vi "MB Serial Master Query Read HF.vi"(8 "error in":errorcluster, 10 "Set Points":dbl[](array[numeric])=[1.0], 11 "VISA resource name":refnum<visa-resource-name>) -> (0 "error out":errorcluster, 2 "Meter reading":sgl, 3 "VISA resource name out":refnum<visa-resource-name>, 5 "Unit id":i32)   [LabVIEW 2015]
doc: "The master uses this VI to read the slaves input registers. This corresponds to a public function code of 4 in the MODBUS protocol."
uses:
  MB Modbus Command.ctl
panel:
  out "Exception Code":u8 format="%.0x"
  in  "Timeout":u32=500
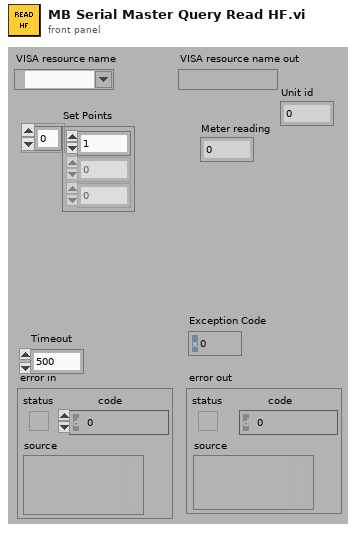
[diagram p1: front panel]
types:
  T1 = typedef "MB Modbus Command.ctl" = cluster{"Function Code":u8, "Starting Address":u16, "Quantity":u16, "Data":u16[], "Discrete":bool[]}
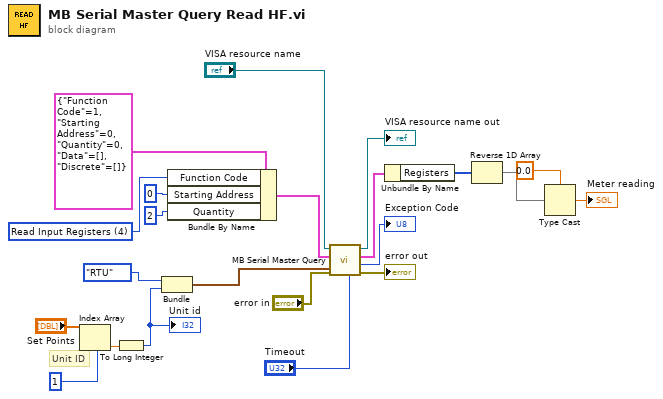
[diagram p0: block diagram]
diagram:
  w19 = u8 4 items=["Read Coils"=1, "Read Discrete Inputs"=2, "Read Holding Registers"=3, "Read Input Registers"=4, "Write Single Coil"=5, "Write Single Register"=6, "Read Exception Status"=7, "Write Multiple Coils"=15, "Write Multiple Registers"=16] ("Function Code")
  # "Unit ID"
  n1 = Index Array(array="Set Points", index=1) -> (element=w2:dbl)
  n2 = To Long Integer(number=w2) -> (32bit integer=w3:i32)
  "Unit id" <- w3
  n3 = Bundle("Mode"=enum16{"RTU", "ASCII"}."RTU", w3) -> (w1:cluster{"Mode":enum16{"RTU", "ASCII"}, i32})  [unwired: 1 in]
  n4 = Bundle By Name(cluster=T1 {"Function Code"=1, "Starting Address"=0, "Quantity"=0, "Data"=[], "Discrete"=[]} ("Modbus Command"), "Function Code"=w19, "Starting Address"=u16 0, "Quantity"=u16 2) -> (w20:T1)
  n5 = call "MB Serial Master Query.vi"("Timeout"="Timeout", "Serial Parameters"=w1, "error in (no error)"="error in", "Modbus Command"=w20, "VISA resource name"="VISA resource name") -> ("error out"=→"error out":errorcluster, "Exception Code"=→"Exception Code":u8, "Registers"=w11:cluster{"Registers":u16[], "Discrete":bool[]}, "VISA resource name out"=→"VISA resource name out":refnum<visa-resource-name>)  [unwired: 2 in, 1 out]
  n6 = Unbundle By Name(w11) -> ("Registers"=w8:u16[])
  n7 = Reverse 1D Array(array=w8) -> (reversed array=w7:u16[])
  n8 = Type Cast(type=sgl 0.0, x=w7) -> (*(type *) &x=→"Meter reading":sgl)
